vi "Matrix RGB FIFO.vi"() -> ()   [LabVIEW 2019]
uses:
  LED Matrix Host/Public/Controls/Animation.ctl
  <vilib>/FPGAPlugInAG/myRIO-1900/niLvFpga_Open_myRIO-1900.vi
  <vilib>/rvi/interface/common/dynamic/niFpgaDynamicAddResources.vi
  <vilib>/Utility/error.llb/Error Cluster From Error Code.vi
  <vilib>/rvi/errors/niLvFpgaAdjustHostInterfaceError.vi
  <vilib>/FPGAPlugInAG/Dynamic/niLvFpga_Close_Dynamic.vi
  <vilib>/rvi/interface/nirviOpenFPGA/nirviOpenFPGA.xnode
  FPGA Bitfiles/ledmatrix_FPGATarget_TestNeopixel_PKs3K1VqgjY.lvbitx
  <vilib>/rvi/interface/nirviMethod/nirviMethod.xnode
  <vilib>/rvi/interface/nirviReadWriteControl/nirviReadWriteControl.xnode
  <vilib>/rvi/interface/nirviCloseFPGA/nirviCloseFPGA.xnode
  LED Matrix Host/LED Matrix Host.lvlib
  NiFpgaLv.dll
  <vilib>/rvi/interface/Simulation/niFpgaSimulationCallBeginRW.vi
  <vilib>/FPGAPlugInAG/Dynamic/niLvFpga_WriteFifo_Dynamic.vi
  <vilib>/rvi/errors/niLvFpgaMergeErrorWithErrorCode.vi
panel:
  out "Empty Elements Remaining":u32
  in  "Color Box":u32(colorbox)=6618880
  in  "Tab Control":enum32{"Matrix Manual", "Animation", "Control"}(tab)
  in  "Matrix":u32[][](array[colorbox])
  in  "Animation":T1
  in  "Tank":u8(slide) max=8 scale=0.0..8.0
  in  "FPS":u32(slide) scale=0.0..100.0
  in  "Update":bool
  in  "stop":bool
  in  "Intensity":sgl(slide) scale=0.0..1.0
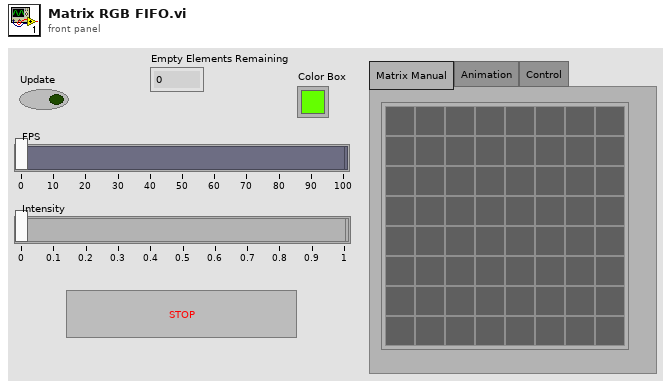
[diagram p1: front panel]
types:
  T1 = typedef "LED Matrix Host.lvlib/Animation.ctl" = enum16{"Pixel Pass", "Columns Pass", "Rows Pass", "Frame Pass"}
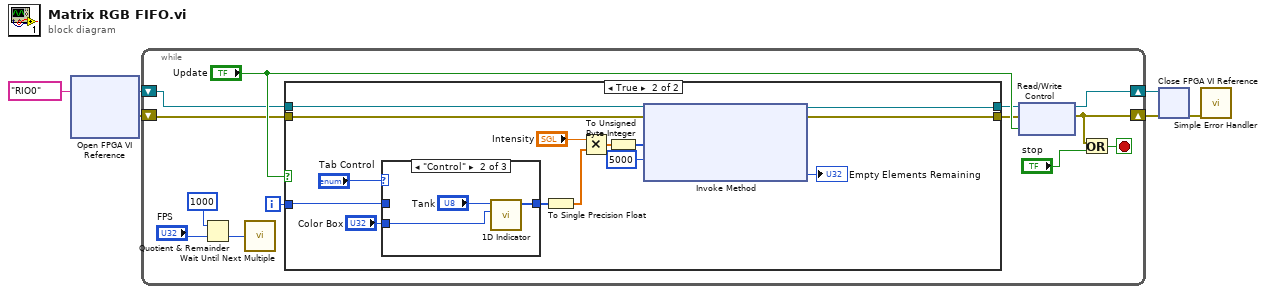
[diagram p0: block diagram]
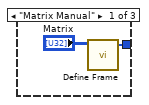
[diagram p3: hidden frame]
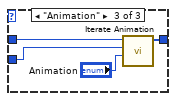
[diagram p4: hidden frame]
diagram:
  n1 = xnode "Open FPGA VI Reference"("resource name"=tag "RIO0") -> ("FPGA VI Reference Out"=w5:refnum<k20>, "error out"=w4:errorcluster)  [unwired: 1 in]
  n2 = while {
    shift-right: [w10] -> w3
    shift-left: w5 -> [w14]
    shift-right: [w9] -> w2
    shift-left: w4 -> [w13]
    i -> [w15]
    stop <- w8 stop-if-true
    n3 = Quotient & Remainder(x=u32 1000 ("y"), y="FPS") -> (floor(x/y)=w17:u32)  [unwired: 1 out]
    n4 = call "Wait Until Next Multiple"("Count(mSec)"=w17) -> ()  [unwired: 1 out]
    n5 = case shown="True" "Update" {
      tunnel: w15 -> [_ w24]
      tunnel: w14 -> [w21 w29]
      tunnel: w13 -> [w20 w28]
      tunnel: [w20 w26] -> w12
      tunnel: [w21 w25] -> w11
      frame False {
      }
      frame True {
        n6 = case shown="\"Control\"" "Tab Control" {
          tunnel: [w37 w38 w44] -> w32
          tunnel: w24 -> [_ _ w43]
          tunnel: "Color Box" -> [_ w39 w41]
          frame "Matrix Manual" {
            n7 = call "Define Frame.vi"("Matrix"="Matrix") -> ("Array"=w37:u8[])  [unwired: 10 in]
          }
          frame "Control" {
            n8 = call "1D Indicator.vi"("Color"=w39, "Numeric Value"="Tank") -> ("Raw Data"=w38:u8[])  [unwired: 9 in]
          }
          frame "Animation" {
            n9 = call "Iterate Animation.vi"("Animation"="Animation", "Color"=w41, "Index"=w43) -> ("Raw Data"=w44:u8[])  [unwired: 8 in]
          }
        }
        n10 = To Single Precision Float(number=w32) -> (single precision float=w33:sgl[])
        n11 = Multiply(x="Intensity", y=w33) -> (x*y=w34:sgl[])
        n12 = To Unsigned Byte Integer(number=w34) -> (unsigned 8bit integer=w27:u8[])
        n13 = xnode "Invoke Method"("FPGA VI Reference In"=w29, "error in"=w28, "Data"=w27, "Timeout (ms)"=5000) -> ("FPGA VI Reference Out"=w25:refnum<k20>, "error out"=w26:errorcluster, "Empty Elements Remaining"=→"Empty Elements Remaining":u32)
      }
    }
    n14 = xnode "Read/Write Control"("FPGA VI Reference In"=w11, "error in"=w12, "Update"="Update") -> ("FPGA VI Reference Out"=w10:refnum<k20>, "error out"=w9:errorcluster)
    n15 = Or(x=w9, y="stop") -> (x .or. y?=w8:bool)
  }
  n16 = xnode "Close FPGA VI Reference"("FPGA VI Reference In"=w3, "error in"=w2) -> ("error out"=w1:errorcluster)
  n17 = call <vilib>:"Simple Error Handler.vi"("error in (no error)"=w1) -> ()  [unwired: 4 in, 5 out]
